vi "stageMove.vi"(2 "counts/um":dbl=1.0, 3 "position (um)":dbl) -> (0 "error out":errorcluster, 1 "function return":i32)   [LabVIEW 2017]
uses:
  globalDevices.vi
  Stage/ximcLVx64/libximc.lvlib
panel:
  out "stage ids":cluster{"opaque pointer":u64, "id":i32}
  out "error in":errorcluster
  # "IN"
  # "OUT"
  # "STATIC CONFIG"
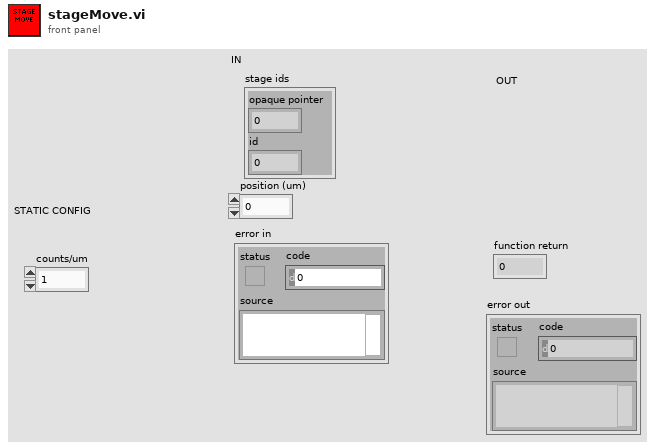
[diagram p1: front panel]
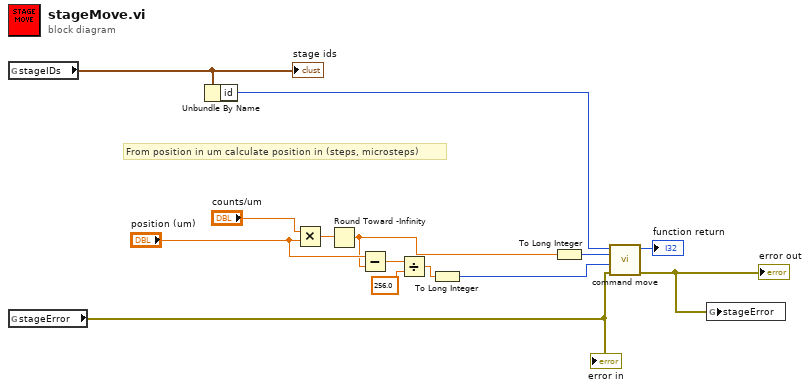
[diagram p0: block diagram]
diagram:
  # "From position in um calculate position in (steps, microsteps)"
  n1 = global read "globalDevices.vi" "stageIDs"() -> (w3:cluster{"opaque pointer":u64, "id":i32})
  "stage ids" <- w3
  n2 = global read "globalDevices.vi" "stageError"() -> (w2:errorcluster)
  "error in" <- w2
  n3 = Unbundle By Name(w3) -> ("id"=w5:i32)
  n4 = Multiply(x="counts/um", y="position (um)") -> (x*y=w12:dbl)
  n5 = Round Toward -Infinity(1:w12) -> (0:w10:dbl)
  n6 = Subtract(x="position (um)", y=w10) -> (x-y=w9:dbl)
  n7 = Divide(x=w9, y=256.0) -> (x/y=w7:dbl)
  n8 = To Long Integer(number=w7) -> (32bit integer=w4:i32)
  n9 = To Long Integer(number=w10) -> (32bit integer=w14:i32)
  n10 = call "command move.vi"("error in (no error)"=w2, "uPosition"=w4, "Position"=w14, "id"=w5) -> ("error out"=w1:errorcluster, "function return"=→"function return":i32)  [unwired: 6 in]
  "error out" <- w1
  n11 = global write "globalDevices.vi" "stageError"(w1) -> ()
